vi "New Node On Wire_HELPER.vi"(2 "Variant In 2":variant, 4 "Variant In 1":variant) -> (1 "Variant Out 2":variant, 5 "Variant Out 1":variant)   [LabVIEW 2023]
panel:
  # "This wiring pattern attempts to keep a vertical wire inplace when we insert this VI on the wire. We also have a backwards (in on right, out on left) set of terminals, for the rare case where a wire is going the wrong way.\n\nThere will be a small offset for wires going up. We could fix this if we really wanted to"
  # "VI has no icon so it doesn't appear during scripting operations"
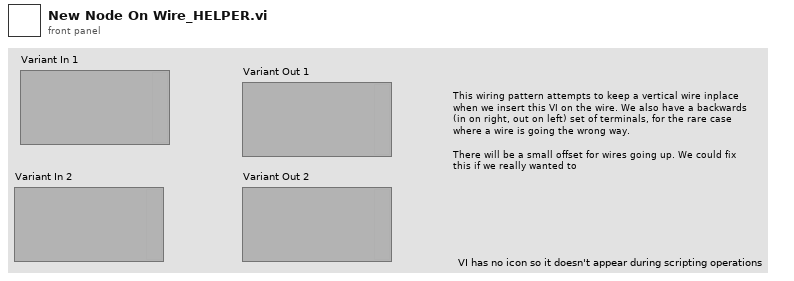
[diagram p1: front panel]
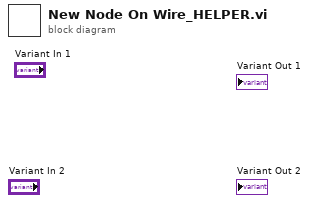
[diagram p0: block diagram]
diagram:
